vi "completeCycle.vi"(8 "error in (no error)":errorcluster, 11 "PreconditioningMonitor in":refnum<class "PreconditioningMonitor.lvclass">) -> (0 "error out":errorcluster, 1 "preconditioningCycle":u32, 2 "preconditiongCompleteIsTrue":bool, 3 "PreconditioningMonitor out":refnum<class "PreconditioningMonitor.lvclass">)   [LabVIEW 2015, in "PreconditioningMonitor.lvclass"]
uses:
  PreconditioningMonitor.lvclass
  PreconditioningMonitor.lvclass/PreconditioningMonitor.ctl
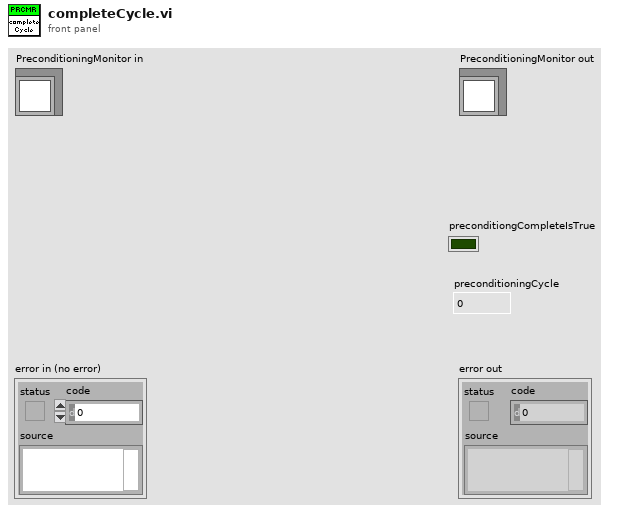
[diagram p1: front panel]
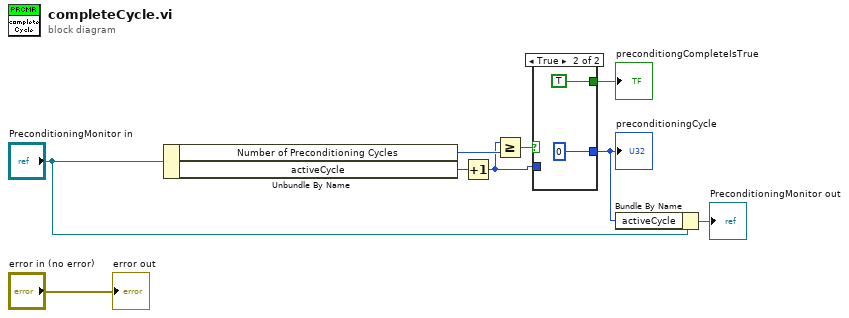
[diagram p0: block diagram]
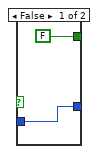
[diagram p2: hidden frame]
diagram:
  n1 = Unbundle By Name("PreconditioningMonitor in") -> ("Number of Preconditioning Cycles"=w5:u32, "activeCycle"=w6:u32)
  n2 = Increment(x=w6) -> (x+1=w2:u32)
  n3 = Greater Or Equal?(x=w2, y=w5) -> (x >= y?=w4:bool)
  n4 = case shown="True" w4 {
    tunnel: [FALSE TRUE] -> w3
    tunnel: w2 -> [w10 _]
    tunnel: [w10 u32 0] -> w1
    frame False {
    }
    frame True {
    }
  }
  "preconditiongCompleteIsTrue" <- w3
  "preconditioningCycle" <- w1
  n5 = Bundle By Name(cluster="PreconditioningMonitor in", "activeCycle"=w1) -> (→"PreconditioningMonitor out":refnum<class "PreconditioningMonitor.lvclass">)
  "error out" <- "error in (no error)"
